vi "Set Trigger Output.vi"(8 "error in (no error)":errorcluster, 10 "Trigger Output (0: Off)":u32(ring) items=["Off", "Div 1", "Div 10", "Div 100"], 11 "VISA resource name":refnum<visa-resource-name>) -> (0 "error out":errorcluster, 3 "VISA resource name out":refnum<visa-resource-name>)   [LabVIEW 2014, in "Fluke 5XXX Series Multicalibrators.lvlib"]
doc: "This VI programs the oscilloscope’s trigger output BNC.\n\nNote:\n\nThis VI is available only for instrument models 5500A and 5520A with oscilloscope option SC300 (SC600 or SC1100)."
uses:
  Fluke 5XXX Series Multicalibrators.lvlib
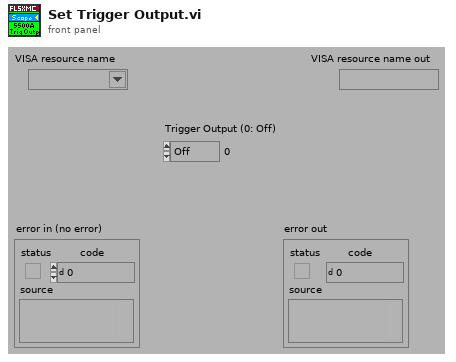
[diagram p1: front panel]
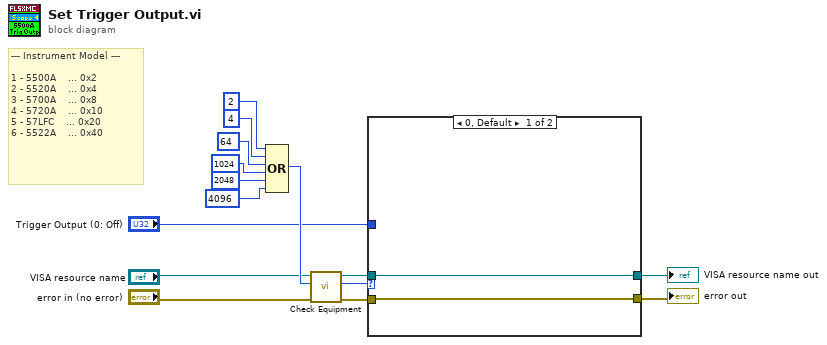
[diagram p0: block diagram]
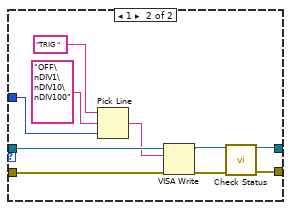
[diagram p2: hidden frame]
diagram:
  # "--- Instrument Model ---\n\n1 - 5500A    ... 0x2\n2 - 5520A    ... 0x4\n3 - 5700A    ... 0x8\n4 - 5720A    ... 0x10\n5 - 57LFC    ... 0x20\n6 - 5522A    ... 0x40"
  n1 = Compound Arithmetic op=OR(2 ("Numeric"), 4 ("Numeric"), 64 ("Numeric"), 1024 ("Numeric"), 2048 ("Numeric"), 4096 ("Numeric")) -> (w8:i32)
  n2 = call "Check Equipment.vi"("error in (no error)"="error in (no error)", "Bit Mask"=w8, "VISA resource name"="VISA resource name") -> ("error out"=w11:errorcluster, "Present?"=w10:u32, "VISA resource name out"=w9:refnum<visa-resource-name>)  [unwired: 6 in]
  n3 = case shown="0, Default" w10 {
    tunnel: "Trigger Output (0: Off)" -> [_ w22]
    tunnel: [w16 w18] -> w6
    tunnel: w11 -> [w17 w25]
    tunnel: w9 -> [w16 w24]
    tunnel: [w17 w21] -> w7
    frame 0, Default {
    }
    frame 1 {
      n4 = Pick Line(string ("")="TRIG " ("Reset Command"), multi-line string="OFF\nDIV1\nDIV10\nDIV100", line index=w22) -> (output string=w23:string)
      n5 = VISA Write(VISA resource name=w24, write buffer=w23, error in (no error)=w25) -> (VISA resource name out=w19:refnum<visa-resource-name>, error out=w20:errorcluster)  [unwired: 1 out]
      n6 = call "Check Status.vi"("VISA resource name"=w19, "error in (no error)"=w20) -> ("VISA resource name out"=w18:refnum<visa-resource-name>, "error out"=w21:errorcluster)  [unwired: 12 in]
    }
  }
  "VISA resource name out" <- w6
  "error out" <- w7
